vi "Write Serial Device.lvclass.vi"(8 "error in (no error)":errorcluster, 10 "Serial Device.lvclass":refnum<class "Serial Device.lvclass">, 11 "UI ACTOR in":refnum<class "UI ACTOR.lvclass">) -> (0 "error out":errorcluster, 3 "UI ACTOR out":refnum<class "UI ACTOR.lvclass">)   [LabVIEW 2020, in "UI ACTOR.lvlib" / "UI ACTOR.lvclass"]
uses:
  UI ACTOR.lvclass
  HAL/Proyecto-Final/Abstract/Serial Device/Serial Device.lvclass
  UI ACTOR.lvclass/UI ACTOR.ctl
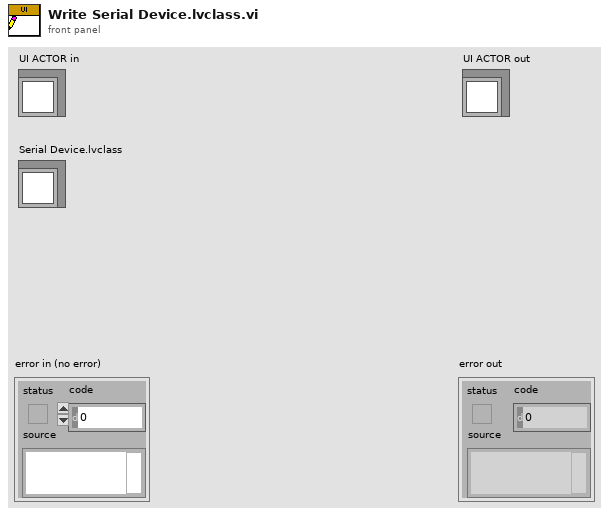
[diagram p1: front panel]
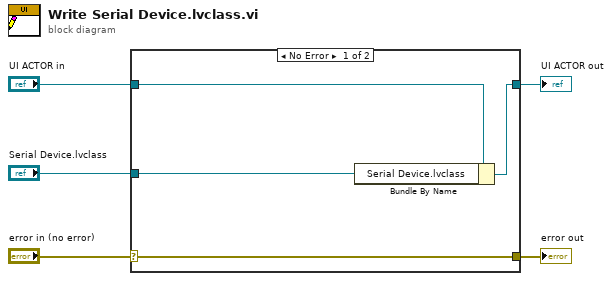
[diagram p0: block diagram]
diagram:
  n1 = case shown="No Error" "error in (no error)" {
    selector: "error in (no error)" -> [w9 w10]
    tunnel: [w9 w10] -> w4
    tunnel: [w7 w11] -> w2
    tunnel: "UI ACTOR in" -> [w8 w11]
    tunnel: "Serial Device.lvclass" -> [w6 _]
    frame No Error {
      n2 = Bundle By Name(cluster=w8, "Serial Device.lvclass"=w6) -> (w7:refnum<class "UI ACTOR.lvclass">)
    }
    frame Error {
    }
  }
  "error out" <- w4
  "UI ACTOR out" <- w2
